vi "ChoiceLineInComboBox(SubVI).vi"(8 "Error In":errorcluster, 10 "ComboBox in":refnum<vi>, 11 "Cluster in":refnum<vi>) -> (0 "Error Out":errorcluster)   [LabVIEW 2018]
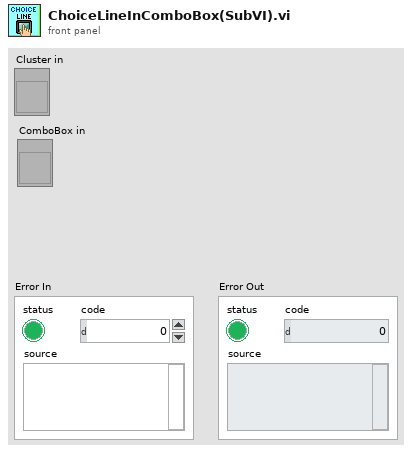
[diagram p1: front panel]
types:
  T1 = typedef "LVComboBoxStrsAndValuesArrayTypeDef.ctl" = cluster{"String":string, "Value":string}[]
  T2 = typedef "STM GRAPH.ctl" = cluster{"Graph settings":T3, "Lines":T4[], "Data":string}
  T3 = typedef "Graph settings.ctl" = cluster{"Axis X Min":dbl, "Axis X Name":string, "Axis X Max":dbl, "Axis Y Min":dbl, " Axis Y Name":string, "Axis Y Max":dbl, "Autoscale":enum16{"Yes", "No", "Only Oy", "Only Ox"}, "Choice Line":dbl}
  T4 = typedef "Line.ctl" = cluster{"Width":dbl, "Color":i64, "Array Oy":dbl[], "Array Ox":dbl[], "Name":string, "Plot Visible":T5}
  T5 = typedef "View.ctl" = bool
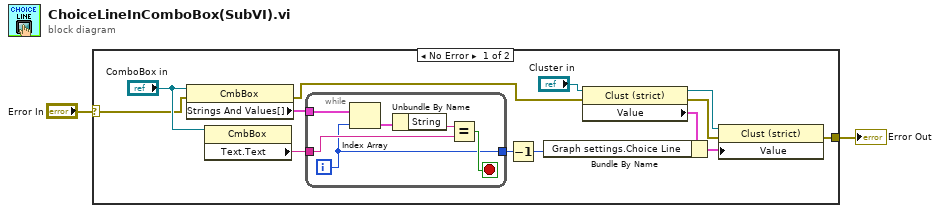
[diagram p0: block diagram]
diagram:
  n1 = case shown="No Error" "Error In" {
    selector: "Error In" -> [w11 w22]
    tunnel: [w3 w22] -> w1
    frame No Error {
      n2 = property on="Property Node" class="CmbBox"(reference="ComboBox in", error in=w11) -> (error out=w5:errorcluster, "Strings And Values[]"=w14:T1)  [unwired: 1 out]
      n3 = property on="Property Node" class="CmbBox"(reference="ComboBox in") -> ("Text.Text"=w13:string)  [unwired: 1 in, 2 out]
      n4 = while {
        tunnel: w14 -> [w21]
        tunnel: w13 -> [w19]
        tunnel: [w16] -> w15
        i -> [w16]
        stop <- w20 stop-if-true
        n5 = Index Array(array=w21, index=w16) -> (element=w18:cluster{"String":string, "Value":string})
        n6 = Unbundle By Name(w18) -> ("String"=w17:string)
        n7 = Equal?(x=w17, y=w19) -> (x = y?=w20:bool)
      }
      n8 = Decrement(x=w15) -> (x-1=w6:i32)
      n9 = property on="Property Node" class="Clust (strict)"(reference="Cluster in", error in=w5) -> (reference out=w10:refnum<vi>, error out=w4:errorcluster, "Value"=w8:T2)
      n10 = Bundle By Name(cluster=w8, "Graph settings.Choice Line"=w6) -> (w9:T2)
      n11 = property on="Property Node" class="Clust (strict)"(reference=w10, error in=w4, "Value"=w9) -> (error out=w3:errorcluster)  [unwired: 1 out]
    }
    frame Error {
    }
  }
  "Error Out" <- w1
